vi "I2C Master.vi"(4 "Configuration":u8, 5 "Counter":u8=187, 6 "Control":u8, 7 "Address In":u8, 8 "SCL_IN":bool, 9 "SDA_IN":bool, 10 "Execute?":T1, 11 "Data Out":u8) -> (0 "SCL_OUT":bool, 1 "SDA_OUT":bool, 2 "Status":u8, 3 "Data In":u8)   [LabVIEW 2017]
doc: "This VI handles the I2C protocol to transfer data between the master and the slave using Serial Data Line (<b>SDA</b>) and Serial Clock Line (<b>SCL</b>)."
uses:
  Utilities/Start Boolean.ctl
  I2C States.ctl
  I2C Status Signals.ctl
panel:
  # "This VI handles the I2C protocol to transfer data between the master and the slave using Serial Data Line (SDA) and Serial Clock Line (SCL).\n \nI2C Configuration:\nBit [7:1] : Reserved\nBit 0     : Enable or Disable I2C functionality\n \nI2C Control:                                                      I2C Status:\nBit [7:4] : Reserved                                           Bit [7:6] : Reserved\nBit 3     : Data Acknowledge Enable               Bit 5     : I2C bus is busy \nBit 2     : Generate the STOP condition          Bit 4     : I2C subsystem is in use\nBit 1     : Generate the START condition        Bit 3     : Data Not Acknowledge received\nBit 0     : Transmit or receive a data type       Bit 2     : Address Not Acknowledge received\n                                                                            Bit 1     : Error\n                                                                       Bit 0     : I2C subsystem is busy"
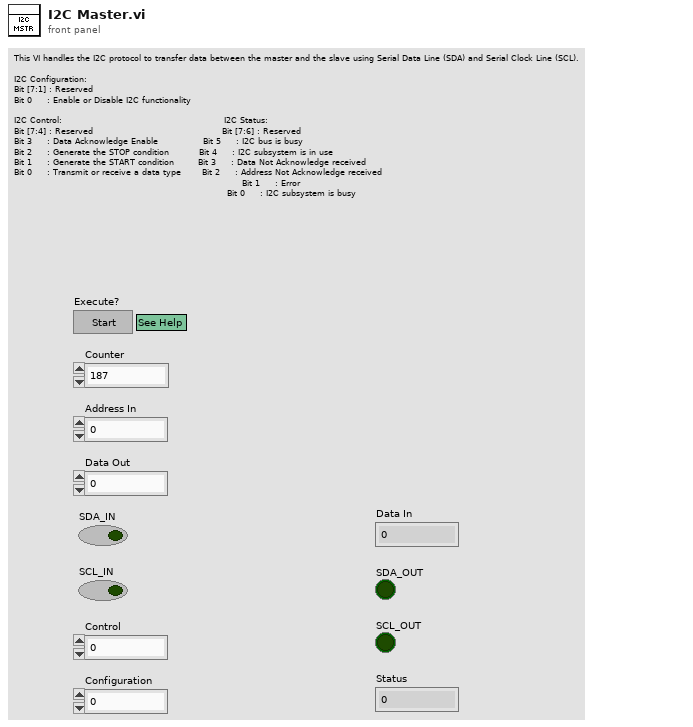
[diagram p1: front panel]
types:
  T1 = typedef "Start Boolean.ctl" = bool
  T2 = typedef "I2C Status Signals.ctl" = cluster{"State":T3, "Timer.Timeout?":bool, "Frame.Complete?":bool, "Data.Address?":bool, "ACK.Address?":bool, "ACK.Stored?":bool}
  T3 = typedef "I2C States.ctl" = fxp<+,5,5>
  T4 = typedef "I2C Configuration.ctl" = cluster{"Enable":bool, "R/S":bool, "Stop":bool, "Start":bool, "Run":bool}
  T5 = typedef "I2C Control Signals.ctl" = cluster{"State+":T3, "Timer.HighPeriod?":bool, "Timer.Load?":bool, "Timer.Increment.":bool, "Frame.LoadSize?":bool, "Frame.Increment":bool, "Data.Address?":bool, "Data.Load":bool, "Data.Setup":bool, "Data.Reset":bool, "Data.Sample":bool, "SDA.Clear":bool, "SDA.Set":bool, "ACK.Sample":bool, "Bus Busy?":bool, "Controller In Use?":bool, "Controller Busy?":bool, "ACK.Store":bool}
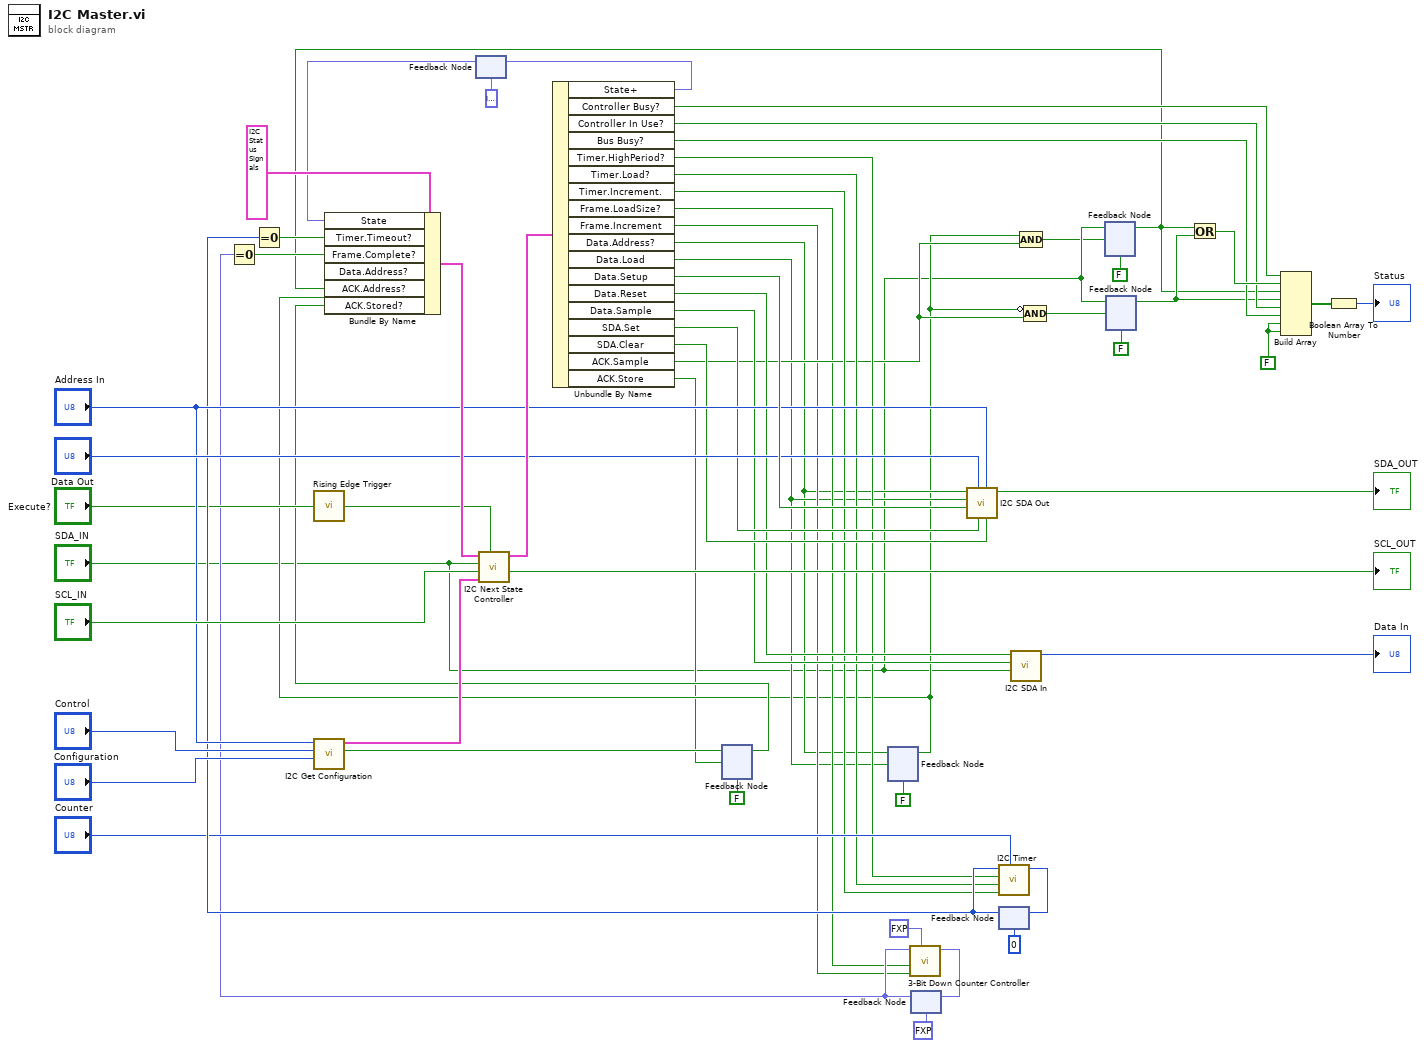
[diagram p0: block diagram]
diagram:
  w40 = FALSE ("element")
  n1 = call "Rising Edge Trigger.vi"("Signal"="Execute?") -> ("Trigger?"=w27:bool)
  n2 = call "I2C Get Configuration.vi"("Configuration"="Configuration", "Control"="Control", "Address In"="Address In") -> ("ACK"=w10:bool, "I2C Configuration"=w22:T4)  [unwired: 7 in]
  n3 = feedback #1(T3 0.0 ("State+")) -> (w55:T3)
  n4 = feedback #2(FALSE ("SDA_IN")) -> (w9:bool)
  n5 = feedback #3(FALSE ("SDA_IN")) -> (w5:bool)
  n6 = feedback #4(fxp<+,3,3> 0.0 ("Input")) -> (w19:fxp<+,3,3>)
  n7 = Equal To 0?(x=w19) -> (x = 0?=w53:bool)
  n8 = feedback #5(u8 0 ("Config 2")) -> (w35:u8)
  n9 = Equal To 0?(x=w35) -> (x = 0?=w54:bool)
  n10 = feedback #6(FALSE ("SDA_IN")) -> (w12:bool)
  n11 = Bundle By Name(cluster=T2 {"State"=0.0, "Timer.Timeout?"=FALSE, "Frame.Complete?"=FALSE, "Data.Address?"=FALSE, "ACK.Address?"=FALSE, "ACK.Stored?"=FALSE} ("Status"), "State"=w55, "Timer.Timeout?"=w54, "Frame.Complete?"=w53, "Data.Address?"=w5, "ACK.Address?"=w12, "ACK.Stored?"=w9) -> (w57:T2)
  n12 = call "I2C Next State Controller.vi"("Execute?"=w27, "I2C Configuration"=w22, "SCL_IN"="SCL_IN", "SDA_IN"="SDA_IN", "Status"=w57) -> ("SCL_OUT"=→"SCL_OUT":bool, "Control"=w56:T5)  [unwired: 5 in]
  n13 = Unbundle By Name(w56) -> ("State+"=w30:T3, "Controller Busy?"=w29:bool, "Controller In Use?"=w25:bool, "Bus Busy?"=w24:bool, "Timer.HighPeriod?"=w31:bool, "Timer.Load?"=w32:bool, "Timer.Increment."=w33:bool, "Frame.LoadSize?"=w18:bool, "Frame.Increment"=w17:bool, "Data.Address?"=w6:bool, "Data.Load"=w7:bool, "Data.Setup"=w48:bool, "Data.Reset"=w36:bool, "Data.Sample"=w37:bool, "SDA.Set"=w38:bool, "SDA.Clear"=w39:bool, "ACK.Sample"=w23:bool, "ACK.Store"=w4:bool)
  n14 = feedback-in #1(w30) -> ()
  n15 = feedback-in #2(w10, w4) -> ()
  n16 = feedback-in #3(w6, w7) -> ()
  n17 = call "3-Bit Down Counter Controller.vi"("Input"=fxp<+,3,3> 7.0, "Decrement?"=w17, "Load?"=w18, "Value"=w19) -> ("Value+"=w20:fxp<+,3,3>)  [unwired: 7 in]
  n18 = feedback-in #4(w20) -> ()
  n19 = call "I2C SDA Out.vi"("Clear?"=w39, "Address In"="Address In", "Set?"=w38, "Data In"="Data Out", "Setup?"=w48, "Load?"=w7, "Address?"=w6) -> ("SDA_OUT"=→"SDA_OUT":bool)  [unwired: 4 in]
  n20 = call "I2C Timer.vi"("Counter Value"="Counter", "Decrement?"=w33, "Load?"=w32, "HighPeriod?"=w31, "Value"=w35) -> ("Value+"=w51:u8)  [unwired: 6 in]
  n21 = feedback-in #5(w51) -> ()
  n22 = call "I2C SDA In.vi"("SDA_IN"="SDA_IN", "Sample"=w37, "Reset"=w36) -> ("Data Out"=→"Data In":u8)  [unwired: 8 in]
  n23 = Compound Arithmetic op=AND(w5, w23) -> (w1:bool)
  n24 = Compound Arithmetic op=AND(invert w5, w23) -> (w2:bool)
  n25 = feedback-in #6("SDA_IN", w1) -> ()
  n26 = feedback #7(FALSE ("SDA_IN")) -> (w15:bool)
  n27 = feedback-in #7("SDA_IN", w2) -> ()
  n28 = Or(x=w12, y=w15) -> (x .or. y?=w26:bool)
  n29 = Build Array(w29, w26, w12, w15, w25, w24, w40, w40) -> (w42:bool[])
  n30 = Boolean Array To Number(Boolean array=w42) -> (number=→"Status":u8)
